vi "MB(RTU)test.vi"() -> ()   [LabVIEW 2017]
doc: "Use this template to build a producer/consumer design pattern with events to produce queue items. Use this design pattern instead of the User Interface Event Handler pattern for user interfaces when you want to execute code asynchronously in response to an event without slowing the user interface responsiveness."
uses:
  Controls/SV_MBtest.ctl
  Controls/FV_MBmuster(RTU).ctl
  <vilib>/ErrorRing/Error Ring.xnode
panel:
  in  "Test":bool
  out "register values":u16[](array[numeric])
  in  "holding register values":u16[](array[numeric]) format="%x"
  in  "baud rate (9600)":u32=115200
  in  "VISA resource name":refnum<visa-resource-name>="COM3"
  in  "stop":bool
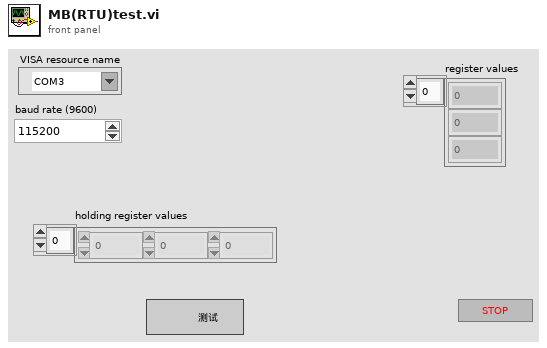
[diagram p1: front panel]
types:
  T1 = typedef "SV_MBtest.ctl" = enum16{"Initialize", "Setup", "Testing", "cleanup"}
  T2 = typedef "FV_MBmuster(RTU).ctl" = enum16{"Initialize", "Create Master", "Write Register", "Read Register", "Close Master"}
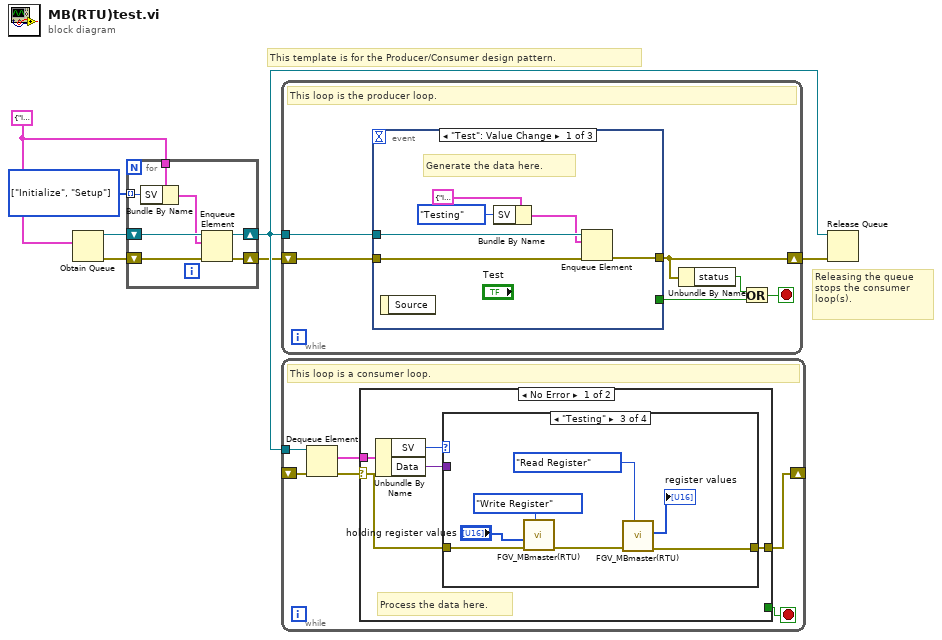
[diagram p0: block diagram]
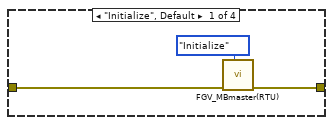
[diagram p2: hidden frame]
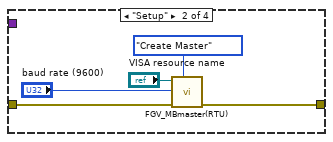
[diagram p3: hidden frame]
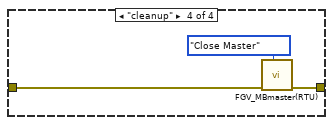
[diagram p4: hidden frame]
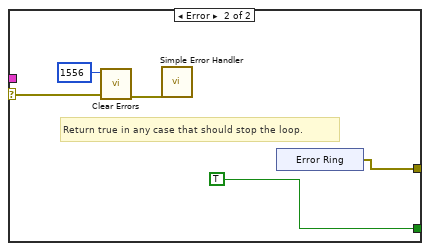
[diagram p5: hidden frame]
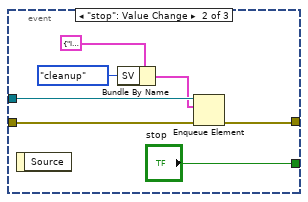
[diagram p6: hidden frame]
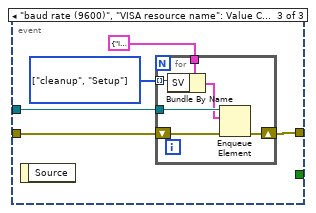
[diagram p7: hidden frame]
diagram:
  w1 = T1[] [enum."Initialize", enum."Setup"] items=["Initialize", "Setup", "Testing", "cleanup"]
  w2 = cluster{"SV":T1, "Data":variant} {"SV"=enum."Initialize", "Data"=variant}
  # "Releasing the queue stops the consumer loop(s)."
  # "This template is for the Producer/Consumer design pattern."
  n1 = Obtain Queue(element data type=w2) -> (queue out=w6:refnum<queue>, error out=w4:errorcluster)  [unwired: 4 in, 1 out]
  n2 = for {
    shift-right: [w13] -> w5
    shift-left: w6 -> [w14]
    shift-right: [w12] -> w3
    shift-left: w4 -> [w11]
    tunnel: w2 -> [w10]
    tunnel: w1 -> [w9] mode=indexing
    n3 = Bundle By Name(cluster=w10, "SV"=w9) -> (w8:cluster{"SV":T1, "Data":variant})
    n4 = Enqueue Element(queue=w14, element=w8, error in (no error)=w11) -> (queue out=w13:refnum<queue>, error out=w12:errorcluster)  [unwired: 1 in, 1 out]
  }
  n5 = while {
    shift-right: [w16] -> w7
    shift-left: w3 -> [w19]
    tunnel: w5 -> [w20]
    stop <- w17 stop-if-true
    # "This loop is the producer loop."
    n6 = event shown="[0] \"Test\": Value Change" {
      selector: _ -> [_ _ _]
      dyn-events: _ -> [_ _ _]
      timeout: _ -> [_ _ _]
      tunnel: w20 -> [w26 w30 w36]
      tunnel: w19 -> [w25 w32 w37]
      tunnel: [w24 w31 w38] -> w16
      tunnel: [_ "stop" _] -> w18
      event "Test": Value Change {
        # "Generate the data here."
        n7 = event-data() -> ()  [unwired: 1 in, 1 out]
        n8 = Bundle By Name(cluster=cluster{"SV":T1, "Data":variant} {"SV"=enum."Initialize", "Data"=variant}, "SV"=SV_MBtest."Testing") -> (w21:cluster{"SV":T1, "Data":variant})
        n9 = Enqueue Element(queue=w26, element=w21, error in (no error)=w25) -> (error out=w24:errorcluster)  [unwired: 1 in, 2 out]
      }
      event "stop": Value Change {
        n10 = event-data() -> ()  [unwired: 1 in, 1 out]
        n11 = Bundle By Name(cluster=cluster{"SV":T1, "Data":variant} {"SV"=enum."Initialize", "Data"=variant}, "SV"=SV_MBtest."cleanup") -> (w27:cluster{"SV":T1, "Data":variant})
        n12 = Enqueue Element(queue=w30, element=w27, error in (no error)=w32) -> (error out=w31:errorcluster)  [unwired: 1 in, 2 out]
      }
      event "baud rate (9600)", "VISA resource name": Value Change {
        w34 = T1[] [enum."cleanup", enum."Setup"] items=["Initialize", "Setup", "Testing", "cleanup"]
        n13 = event-data() -> ()  [unwired: 1 in, 1 out]
        n14 = for {
          tunnel: w36 -> [w42]
          tunnel: cluster{"SV":T1, "Data":variant} {"SV"=enum."Initialize", "Data"=variant} -> [w41]
          shift-right: [w44] -> w38
          shift-left: w37 -> [w43]
          tunnel: w34 -> [w39] mode=indexing
          n15 = Bundle By Name(cluster=w41, "SV"=w39) -> (w40:cluster{"SV":T1, "Data":variant})
          n16 = Enqueue Element(queue=w42, element=w40, error in (no error)=w43) -> (error out=w44:errorcluster)  [unwired: 1 in, 2 out]
        }
      }
    }
    n17 = Unbundle By Name(w16) -> ("status"=w15:bool)
    n18 = Or(x=w15, y=w18) -> (x .or. y?=w17:bool)
  }
  n19 = while {
    tunnel: w5 -> [w50]
    shift-right: [w45] -> _
    shift-left: _ -> [w46]
    stop <- w47 stop-if-true
    # "This loop is a consumer loop."
    n20 = Dequeue Element(queue=w50, error in (no error)=w46) -> (element=w48:cluster{"SV":T1, "Data":variant}, error out=w49:errorcluster)  [unwired: 1 in, 2 out]
    n21 = case shown="No Error" w49 {
      selector: w49 -> [w52 w76]
      tunnel: w48 -> [w55 _]
      tunnel: [_ TRUE] -> w47
      tunnel: [w51 w77] -> w45
      frame No Error {
        # "Process the data here."
        n22 = Unbundle By Name(w55) -> ("SV"=w54:T1, "Data"=w53:variant)
        n23 = case shown="\"Testing\"" w54 {
          tunnel: w53 -> [_ _ _ _]
          tunnel: w52 -> [w57 w61 w70 w72]
          tunnel: [w58 w60 w67 w73] -> w51
          frame "Initialize", Default {
            n24 = call "FGV_MBmaster(RTU).vi"("FV_MBmaster(RTU)"=FV_MBmuster(RTU)."Initialize", "error in (no error)"=w57) -> ("error out"=w58:errorcluster)  [unwired: 8 in, 1 out]
          }
          frame "Setup" {
            n25 = call "FGV_MBmaster(RTU).vi"("FV_MBmaster(RTU)"=FV_MBmuster(RTU)."Create Master", "error in (no error)"=w61, "baud rate (9600)"="baud rate (9600)", "VISA resource name"="VISA resource name") -> ("error out"=w60:errorcluster)  [unwired: 6 in, 1 out]
          }
          frame "Testing" {
            n26 = call "FGV_MBmaster(RTU).vi"("FV_MBmaster(RTU)"=FV_MBmuster(RTU)."Write Register", "error in (no error)"=w70, "holding register values"="holding register values") -> ("error out"=w66:errorcluster)  [unwired: 7 in, 1 out]
            n27 = call "FGV_MBmaster(RTU).vi"("FV_MBmaster(RTU)"=FV_MBmuster(RTU)."Read Register", "error in (no error)"=w66) -> ("error out"=w67:errorcluster, "register values"=→"register values":u16[])  [unwired: 8 in]
          }
          frame "cleanup" {
            n28 = call "FGV_MBmaster(RTU).vi"("FV_MBmaster(RTU)"=FV_MBmuster(RTU)."Close Master", "error in (no error)"=w72) -> ("error out"=w73:errorcluster)  [unwired: 8 in, 1 out]
          }
        }
      }
      frame Error {
        # "Return true in any case that should stop the loop."
        n29 = call <vilib>:"Clear Errors.vi"("error in (no error)"=w76, "specific error code to clear (0: all)"=1556) -> ("error out"=w75:errorcluster)  [unwired: 4 in, 1 out]
        n30 = call <vilib>:"Simple Error Handler.vi"("error in (no error)"=w75) -> ()  [unwired: 4 in, 5 out]
        n31 = xnode "Error Ring"() -> ("error out"=w77:errorcluster)
      }
    }
  }
  n32 = Release Queue(queue=w5, error in (no error)=w7) -> ()  [unwired: 1 in, 3 out]
